vi "myrio_handshake.vi"(0 "VISA resource name":refnum<visa-resource-name>="ASRL1::INSTR", 1 "error in":errorcluster) -> (2 "VISA resource name out":refnum<visa-resource-name>, 3 "error out":errorcluster, 4 "All Clear \nfrom PC?":bool)   [LabVIEW 2014]
panel:
  out "Timeout?":bool
  out "Number of times\nmyRIO has tried to \nListen":i32
  out "GPS 2":cluster{"X pos":i32, "Y pos":i32, "Heading":dbl}
  out "GPS":cluster{"X pos":i32, "Y pos":i32, "Heading":dbl}
  out "Received String\n(2492)":i32
  out "Heard \nNetwork?":bool
  out "Received String\n(1234)":i32
  # "STEP 1"
  # "STEP 3"
  # "STEP 0"
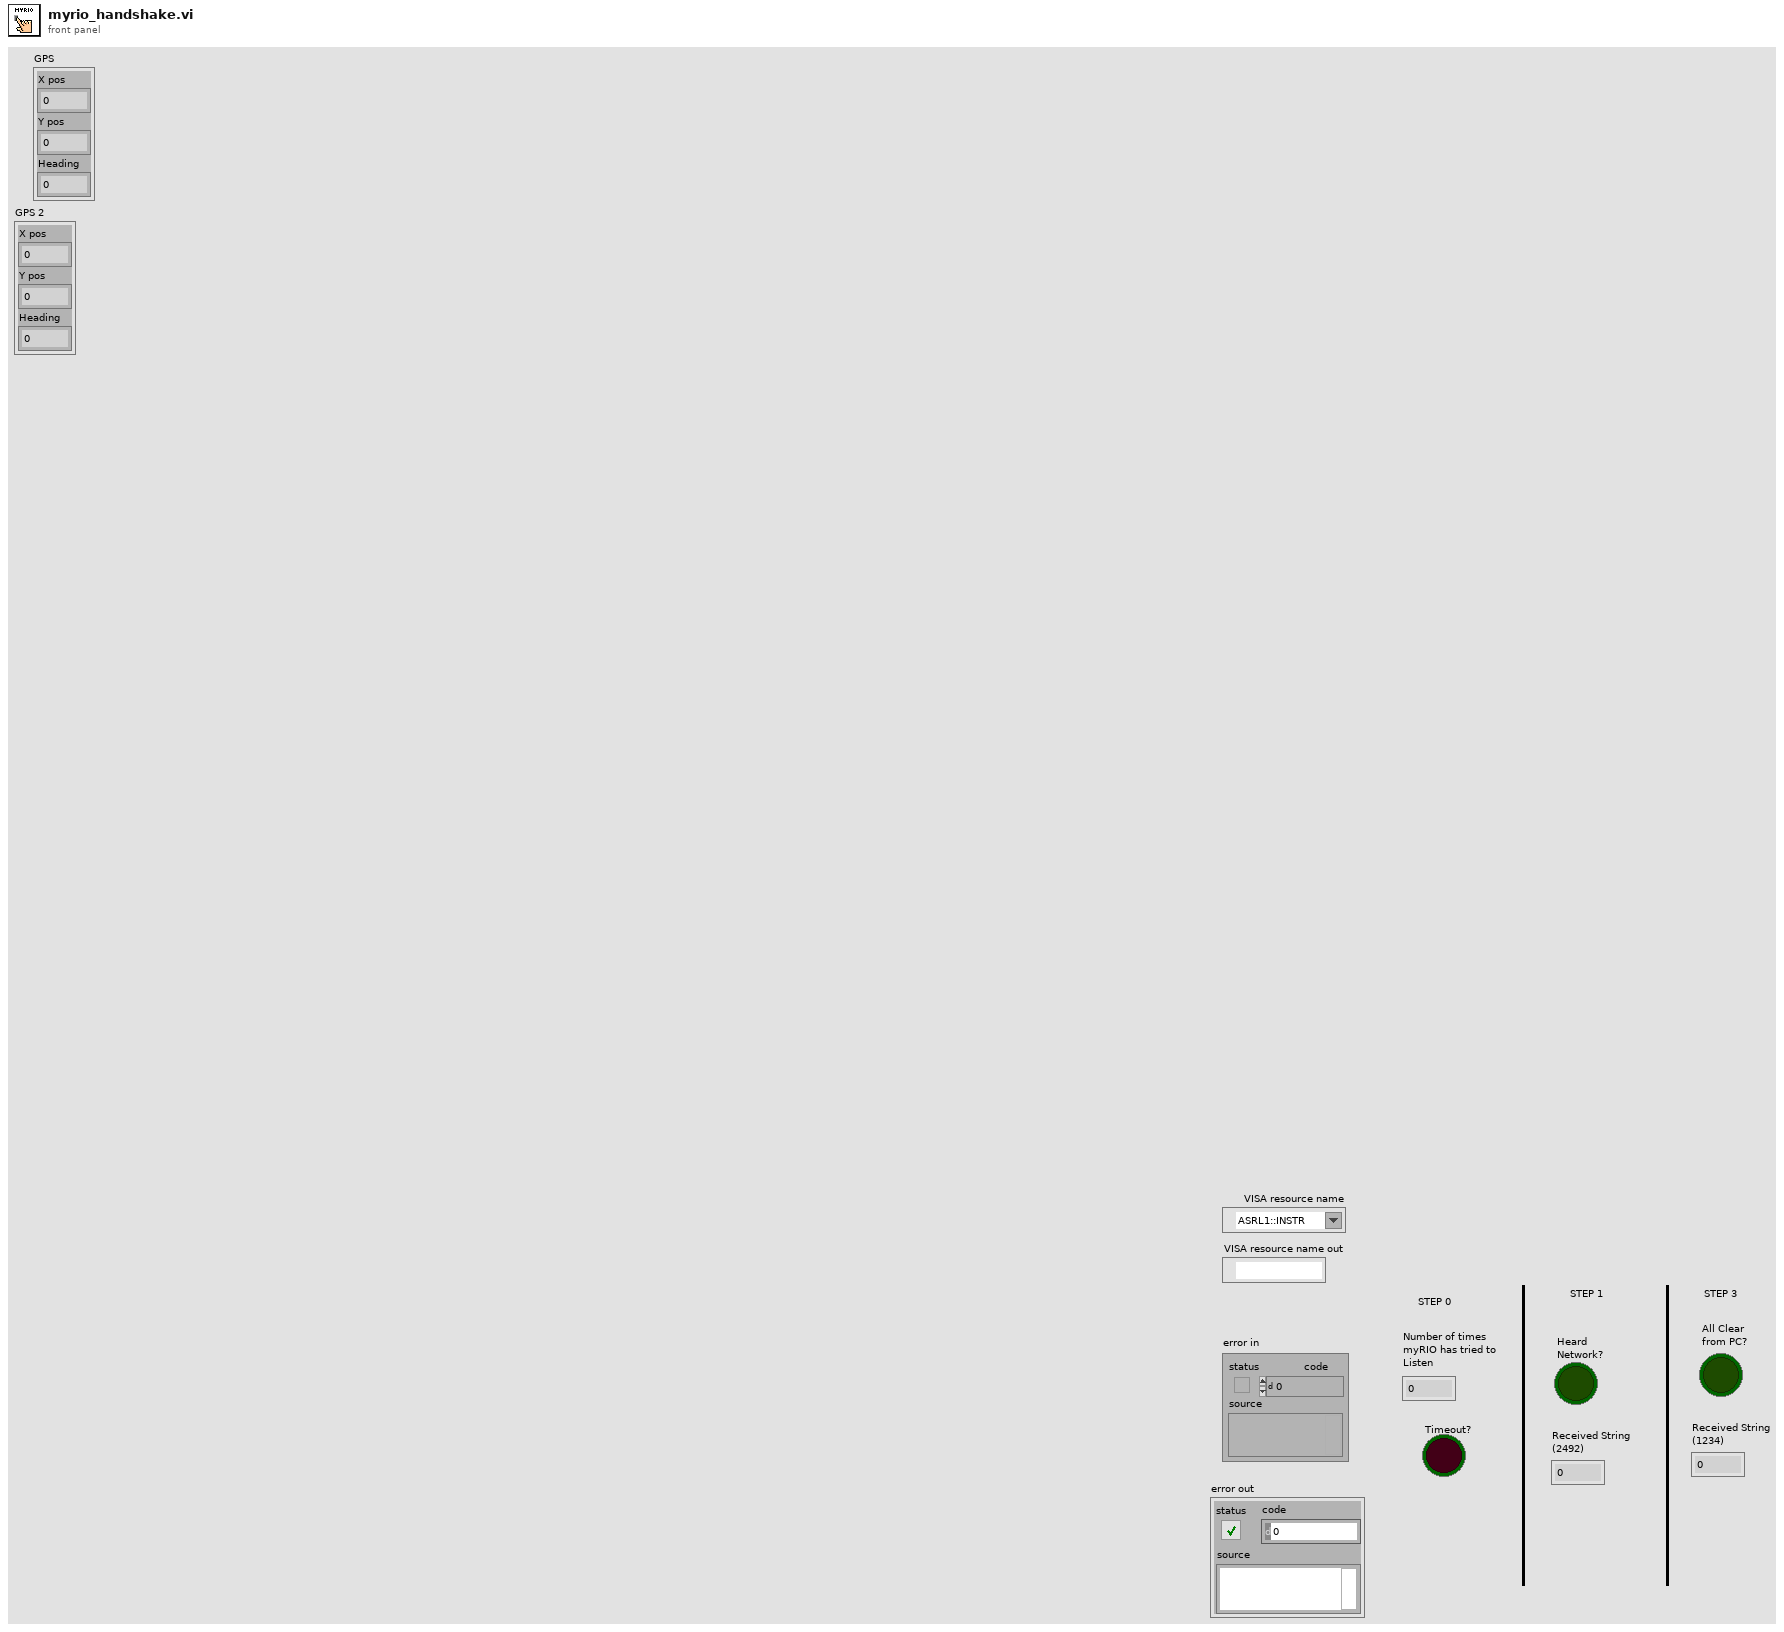
[diagram p1: front panel]
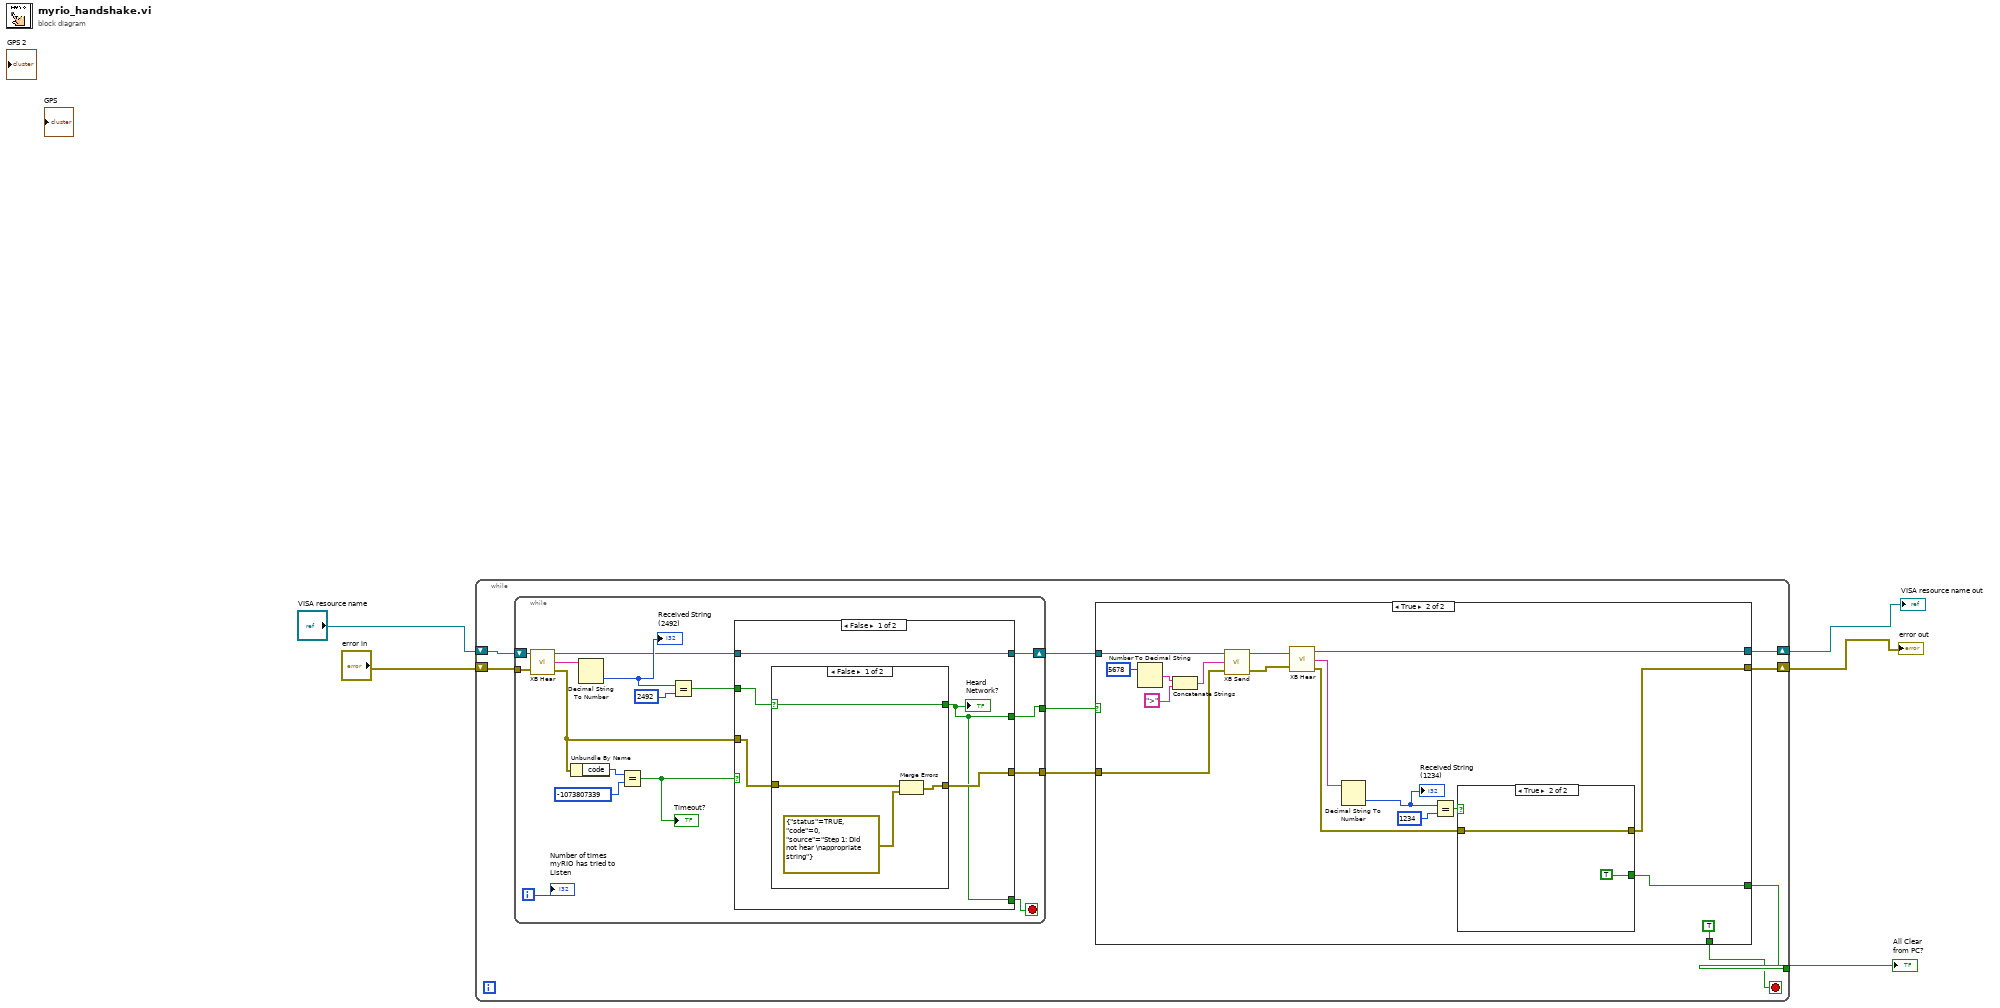
[diagram p0: block diagram]
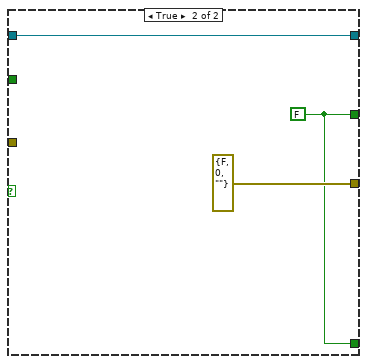
[diagram p3: hidden frame]
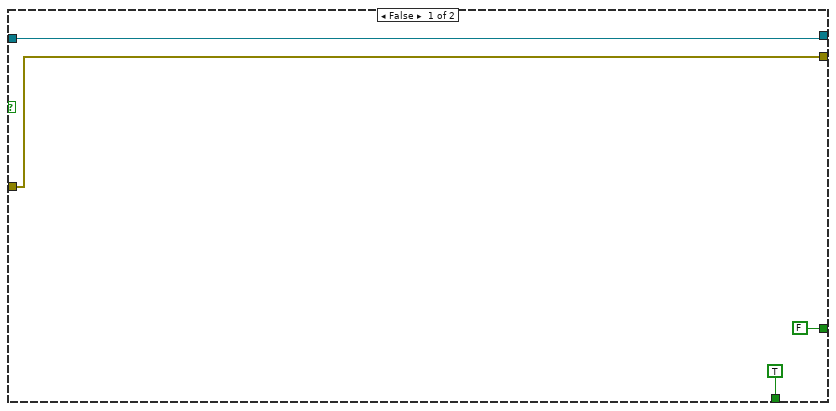
[diagram p4: hidden frame]
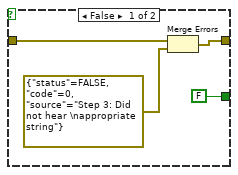
[diagram p5: hidden frame]
diagram:
  n1 = while {
    shift-right: [w14] -> w3
    shift-left: "VISA resource name" -> [w6]
    shift-right: [w12] -> w4
    shift-left: "error in" -> [w7]
    tunnel: [w10] -> w5
    stop <- w9 stop-if-true
    n2 = while {
      tunnel: [w17] -> w11
      shift-right: [w19] -> w8
      shift-left: w6 -> [w24]
      tunnel: w7 -> [w25]
      tunnel: [w30] -> w13
      i -> [w21]
      stop <- w15 stop-if-true
      n3 = call "XB Hear.vi"("VISA resource name"=w24, "error in (no error)"=w25) -> ("VISA resource name out"=w20:refnum<visa-resource-name>, "String Received"=w26:string, "error out"=w18:errorcluster)
      n4 = Unbundle By Name(w18) -> ("code"=w23:i32)
      n5 = Decimal String To Number(string=w26) -> (number=w28:i32)  [unwired: 2 in, 1 out]
      "Received String\n(2492)" <- w28
      n6 = Equal?(x=w23, y=-1073807339) -> (x = y?=w16:bool)
      "Timeout?" <- w16
      n7 = Equal?(x=w28, y=2492) -> (x = y?=w27:bool)
      n8 = case shown="False" w16 {
        tunnel: [w35 errorcluster {"status"=FALSE, "code"=0, "source"=""} ("error IO")] -> w30
        tunnel: w27 -> [w34 _]
        tunnel: w20 -> [w32 w43]
        tunnel: [w32 w43] -> w19
        tunnel: w18 -> [w33 _]
        tunnel: [w31 w42] -> w17
        tunnel: [w31 w42] -> w15
        frame False {
          n9 = case shown="False" w34 {
            selector: w34 -> [w36 w40]
            tunnel: [w37 w41] -> w35
            tunnel: w33 -> [w38 w41]
            tunnel: [w36 w40] -> w31
            frame False {
              n10 = Merge Errors(w38, errorcluster {"status"=TRUE, "code"=0, "source"="Step 1: Did not hear \nappropriate string"} ("error out")) -> (w37:errorcluster)
            }
            frame True {
            }
          }
          "Heard \nNetwork?" <- w31
        }
        frame True {
          w42 = FALSE
        }
      }
      "Number of times\nmyRIO has tried to \nListen" <- w21
    }
    n11 = case shown="True" w11 {
      tunnel: [w47 w65] -> w14
      tunnel: w8 -> [w47 w64]
      tunnel: w13 -> [w48 w63]
      tunnel: [w48 w51] -> w12
      tunnel: [TRUE TRUE] -> w9
      tunnel: [FALSE w50] -> w10
      frame False {
      }
      frame True {
        n12 = Number To Decimal String(number=5678) -> (decimal integer string=w59:string)  [unwired: 1 in]
        n13 = Concatenate Strings(w59, ">" ("string")) -> (w57:string)
        n14 = call "XB Send.vi"("error in (no error)"=w63, "String"=w57, "VISA resource name"=w64) -> ("error out"=w62:errorcluster, "VISA resource name out"=w61:refnum<visa-resource-name>)  [unwired: 1 out]
        n15 = call "XB Hear.vi"("VISA resource name"=w61, "error in (no error)"=w62) -> ("VISA resource name out"=w65:refnum<visa-resource-name>, "String Received"=w56:string, "error out"=w52:errorcluster)
        n16 = Decimal String To Number(string=w56) -> (number=w54:i32)  [unwired: 2 in, 1 out]
        "Received String\n(1234)" <- w54
        n17 = Equal?(x=w54, y=1234) -> (x = y?=w53:bool)
        n18 = case shown="True" w53 {
          tunnel: [w67 w71] -> w51
          tunnel: w52 -> [w68 w71]
          tunnel: [FALSE TRUE] -> w50
          frame False {
            n19 = Merge Errors(w68, errorcluster {"status"=FALSE, "code"=0, "source"="Step 3: Did not hear \nappropriate string"} ("error out")) -> (w67:errorcluster)
          }
          frame True {
          }
        }
      }
    }
  }
  "All Clear \nfrom PC?" <- w5
  "error out" <- w4
  "VISA resource name out" <- w3
